vi "Main Window.vi"() -> ()   [LabVIEW 2020]
uses:
  Control Button/Exit.ctl
  Control Button/login.ctl
  Control Button/Logout.ctl
  Control Button/setting.ctl
  Control Button/report.ctl
  Control Button/Manual.ctl
  Control Button/Start.ctl
  Enqueue/Main window Seq/Test selection_1.ctl
  Enqueue/Main window Seq/Test seq_1.ctl
  Galobal variable_TI.vi
  Project Setup/Globle Variable/GR_Servo.vi
  <vilib>/Utility/file.llb/Read Delimited Spreadsheet (DBL).vi
panel:
  out "Boolean 3":bool
  in  "Boolean 2":bool
  out "Numeric 2":i32
  out "Company Name  2":string
  out "Error":bool
  out "User Name":string
  out "error out":errorcluster
  out "x = y?":bool
  out "Company Name":string
  in  "Sign In":T1
  out "Boolean":bool
  in  "Dashbord":T6
  in  "Login Window":T8 {"User Name" items=["admin", "mmum", "a", "AJAY Kumar", "", "", "", "", "", "", "", "", "", "", "", "", "", "", "", "", "", "", "", "", "", "", "", "", "", "", "", ""]}
  in  "Exit":T9
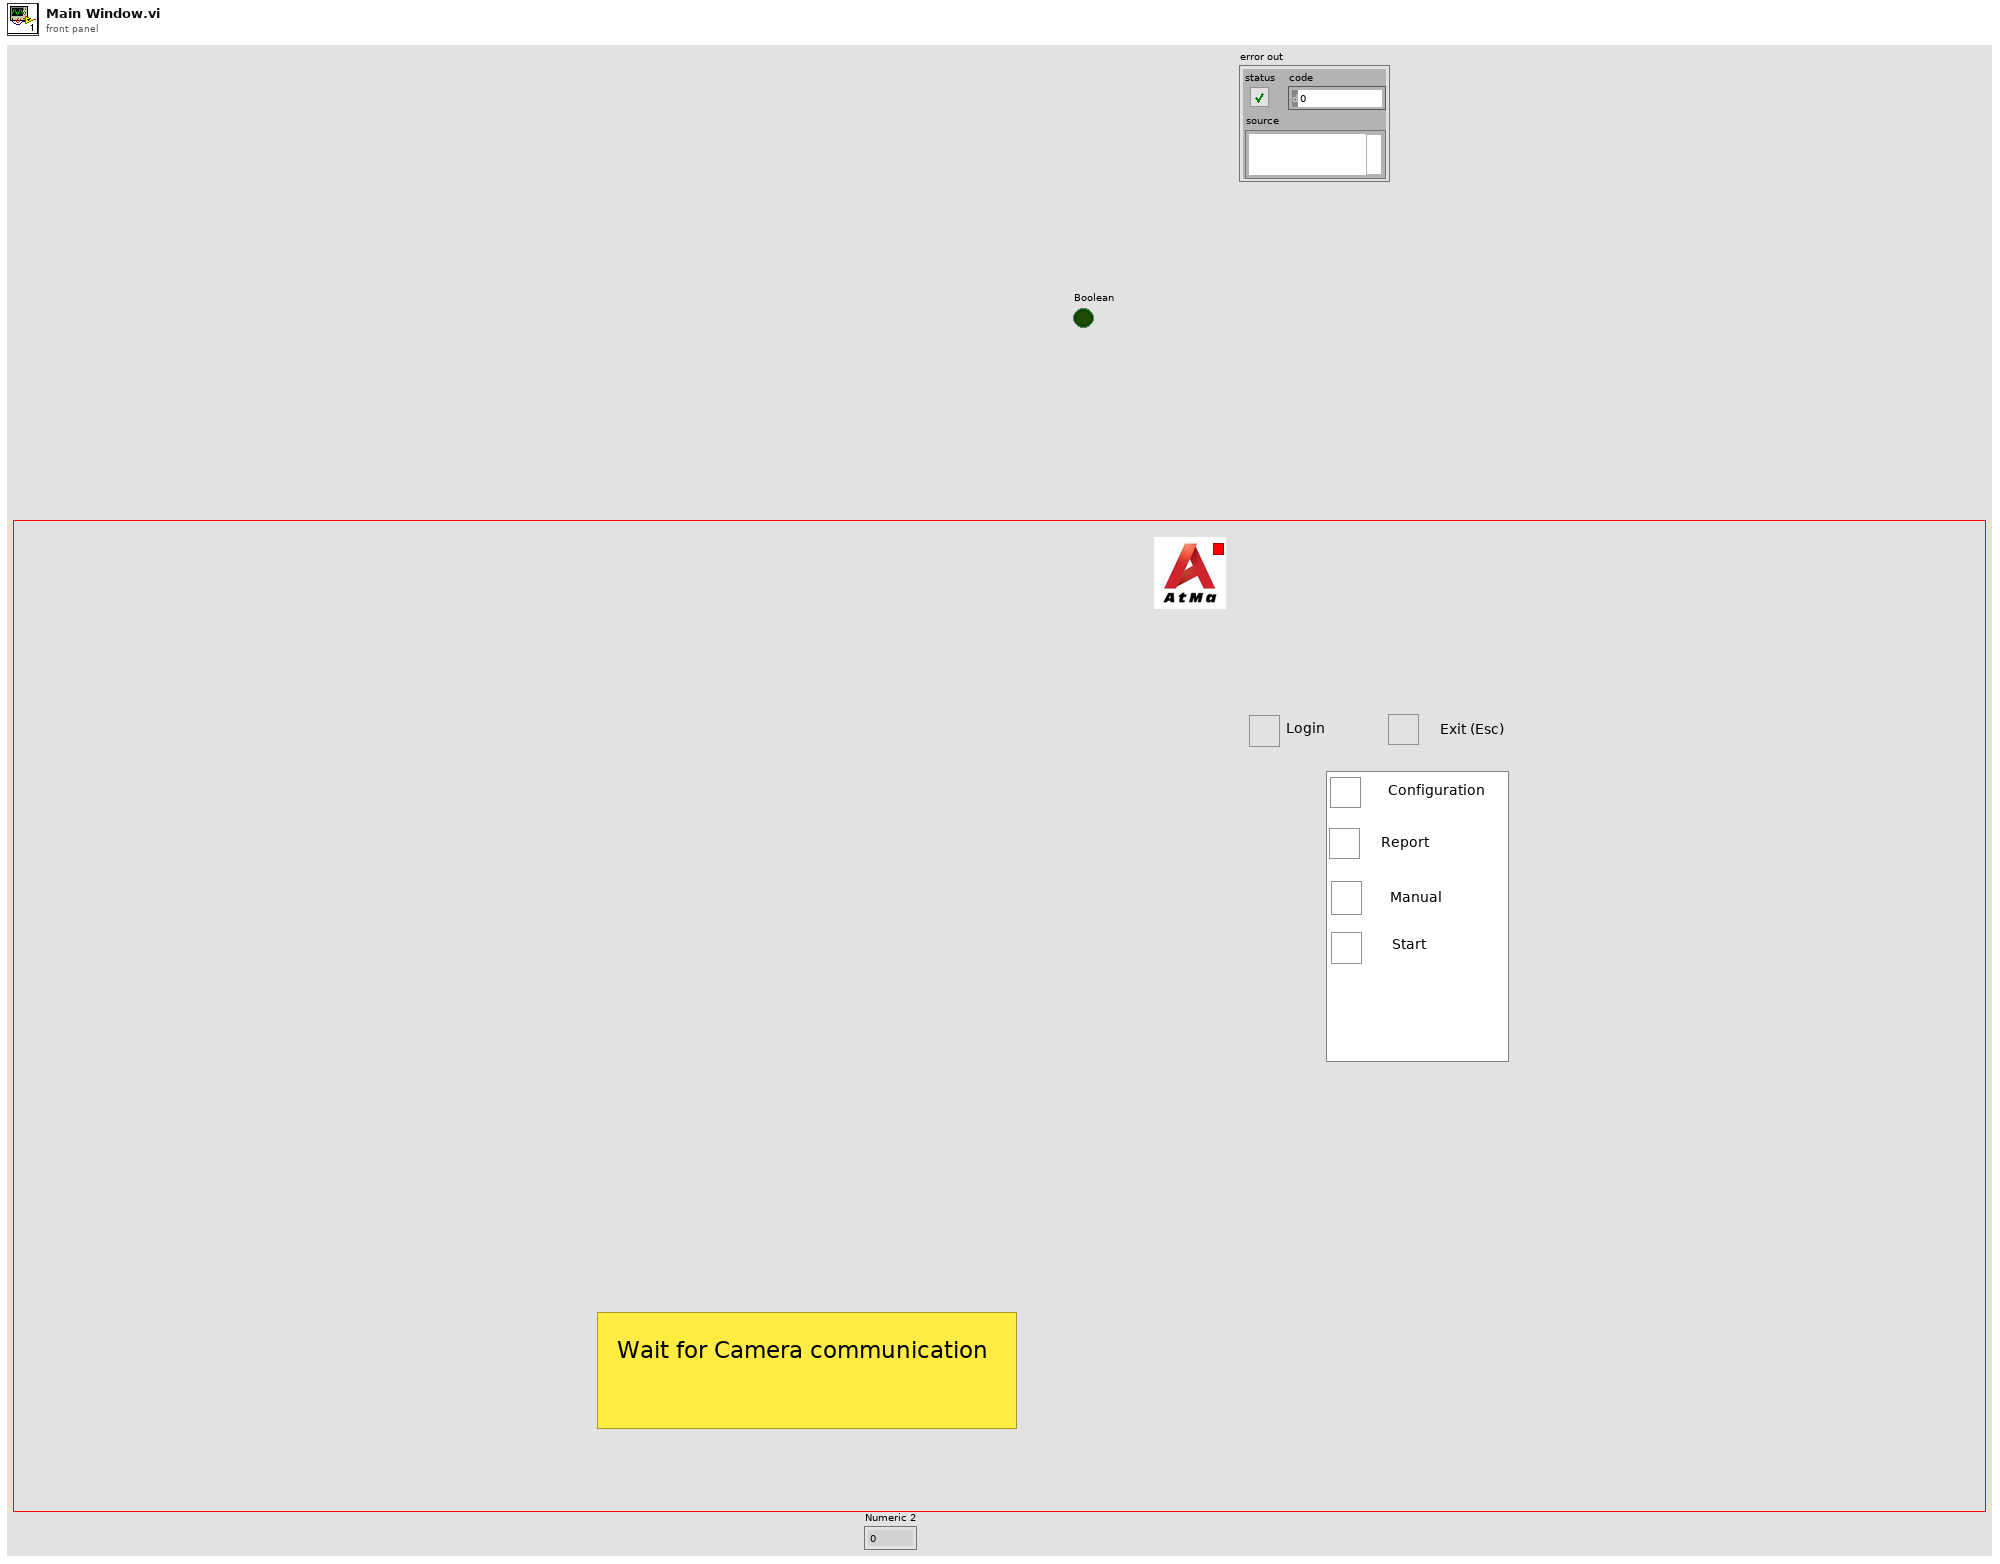
[diagram p1: front panel]
types:
  T1 = typedef "login.ctl" = bool
  T2 = typedef "setting.ctl" = bool
  T3 = typedef "report.ctl" = bool
  T4 = typedef "Manual.ctl" = bool
  T5 = typedef "Start.ctl" = bool
  T6 = cluster{"Setting":T2, "Report":T3, "Manaul":T4, "Start":T5}
  T7 = typedef "Logout.ctl" = bool
  T8 = cluster{"User Name":u16, "Password":string, "Sign In":T1, "Log Out":T7}
  T9 = typedef "Exit.ctl" = bool
  T10 = typedef "Test selection_1.ctl" = enum16{"Init", "Enqueue ", "Enqueue N", "Enqueue in stack", "Enqueue in stack N", "Dequeue", "Dequeue N", "Flush", "Release Queue"}
  T11 = typedef "Test seq_1.ctl" = enum16{"Poll Event", "Login", "Logout", "Confi", "Manual", "Report", "Testing", "Exit"}
  T12 = cluster{"XInput":dbl[], "Y New Value":dbl[], "Avg point":i16}[]
  T13 = cluster{"Slop":dbl[], "Intercept":dbl[], "Average ":i16[]}
  T14 = cluster{"UserName":string[], "Password":string[], "Usertype":string[], "Analog Min":string[], "Analog Max":string[], "DigitalInput Port":string[], "Digital Output Port":string[], "ANalog Port":string[], "IOList":cluster{"DI List_280":string[], "D0List _280":string[], "AI List_280":string[]}}
  T15 = cluster{"DI List_280":string[], "D0List _280":string[], "AI List_280":string[]}
  T16 = cluster{"DigitalInput Port[0]":string, "DigitalInput Port[1]":string, "DigitalInput Port[2]":string, "DigitalInput Port[3]":string, "DigitalInput Port[4]":string, "DigitalInput Port[5]":string, "DigitalInput Port[6]":string, "DigitalInput Port[7]":string, "DigitalInput Port[8]":string, "DigitalInput Port[9]":string, "DigitalInput Port[10]":string, "DigitalInput Port[11]":string, "DigitalInput Port[12]":string, "DigitalInput Port[13]":string, "DigitalInput Port[14]":string, "DigitalInput Port[15]":string}
  T17 = cluster{"Digital Output Port[0]":string, "Digital Output Port[1]":string, "Digital Output Port[2]":string, "Digital Output Port[3]":string, "Digital Output Port[4]":string, "Digital Output Port[5]":string, "Digital Output Port[6]":string, "Digital Output Port[7]":string, "Digital Output Port[8]":string, "Digital Output Port[9]":string, "Digital Output Port[10]":string, "Digital Output Port[11]":string, "Digital Output Port[12]":string, "Digital Output Port[13]":string, "Digital Output Port[14]":string, "Digital Output Port[15]":string, "Digital Output Port[16]":string, "Digital Output Port[17]":string, "Digital Output Port[18]":string, "Digital Output Port[19]":string, "Digital Output Port[20]":string, "Digital Output Port[21]":string, "Digital Output Port[22]":string, "Digital Output Port[23]":string, "Digital Output Port[24]":string, "Digital Output Port[25]":string, "Digital Output Port[26]":string, "Digital Output Port[27]":string, "Digital Output Port[28]":string, "Digital Output Port[29]":string}
  T18 = cluster{"ANalog Port[0]":string, "ANalog Port[1]":string, "ANalog Port[2]":string, "ANalog Port[3]":string, "ANalog Port[4]":string, "ANalog Port[5]":string, "ANalog Port[6]":string, "ANalog Port[7]":string, "ANalog Port[8]":string, "ANalog Port[9]":string, "ANalog Port[10]":string, "ANalog Port[11]":string, "ANalog Port[12]":string, "ANalog Port[13]":string, "ANalog Port[14]":string, "ANalog Port[15]":string, "ANalog Port[16]":string, "ANalog Port[17]":string, "ANalog Port[18]":string, "ANalog Port[19]":string, "ANalog Port[20]":string, "ANalog Port[21]":string, "ANalog Port[22]":string, "ANalog Port[23]":string, "ANalog Port[24]":string, "ANalog Port[25]":string, "ANalog Port[26]":string, "ANalog Port[27]":string, "ANalog Port[28]":string, "ANalog Port[29]":string, "ANalog Port[30]":string, "ANalog Port[31]":string}
  T19 = enum32{"Invalid", "Standard", "Closed", "Hidden", "Minimized", "Maximized"}
  T20 = enum8{"Enabled", "Disabled", "Disabled and Grayed Out"}
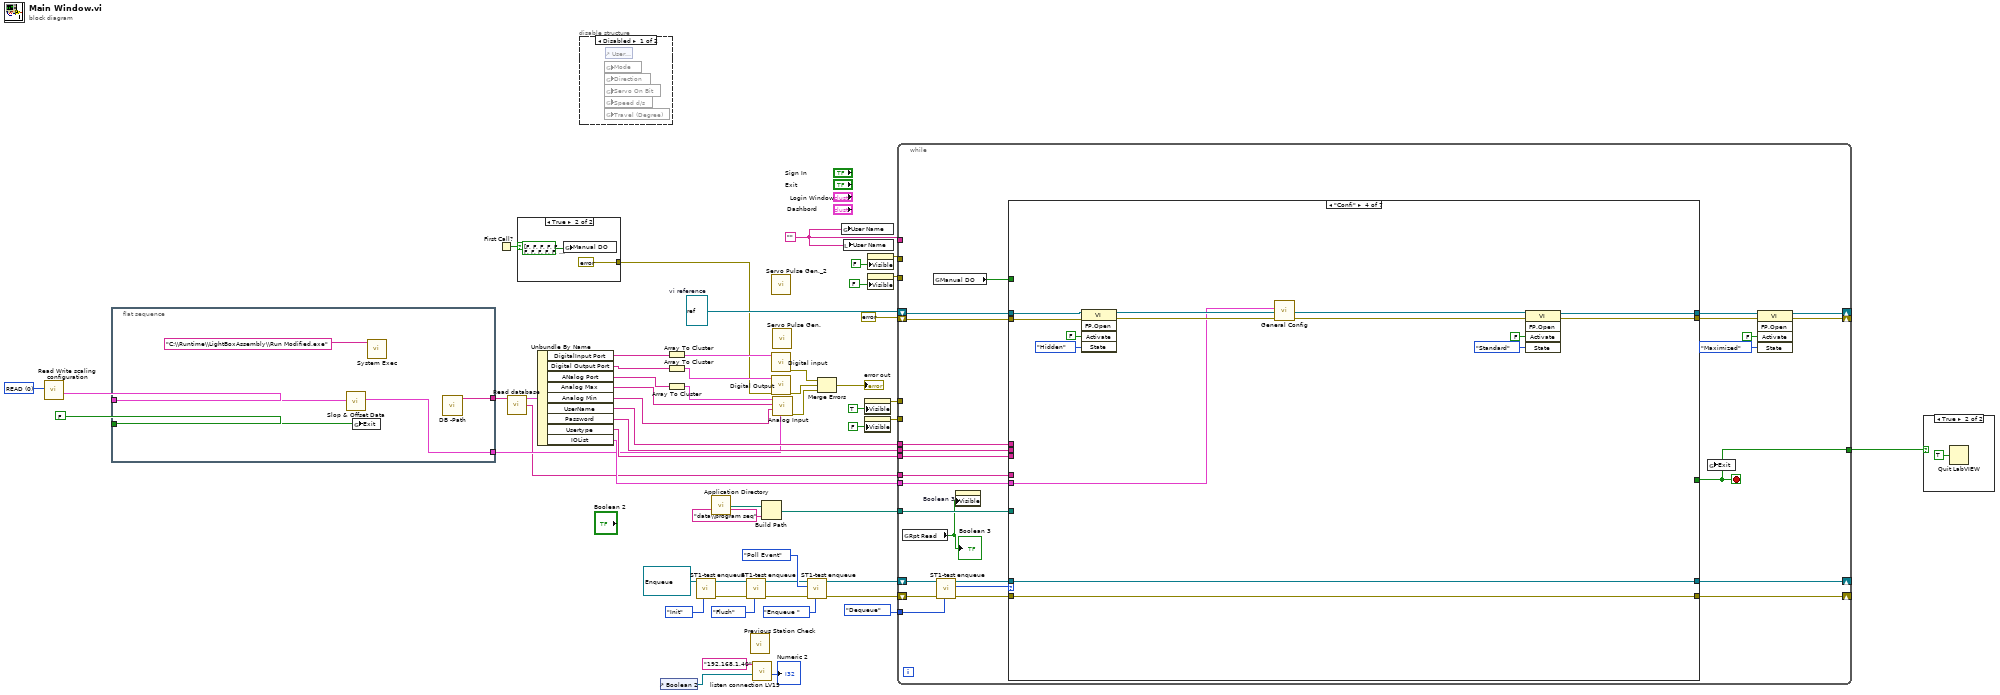
[diagram p0: block diagram]
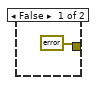
[diagram p3: hidden frame]
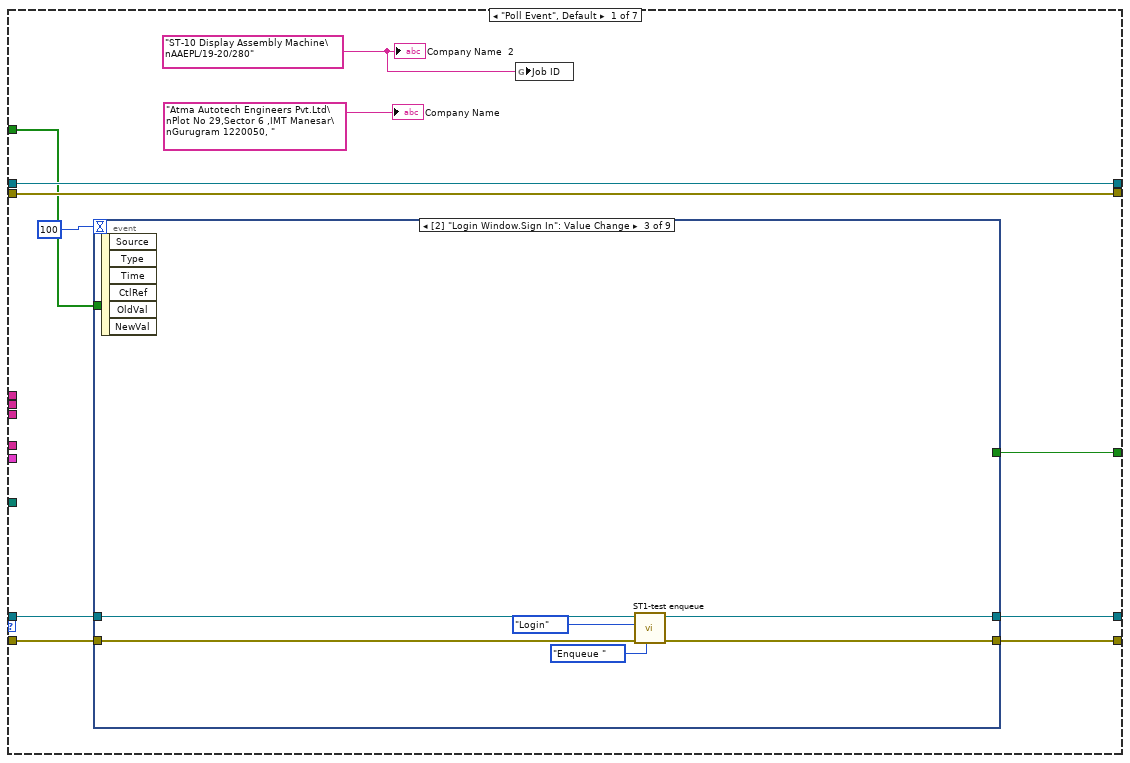
[diagram p5: hidden frame]
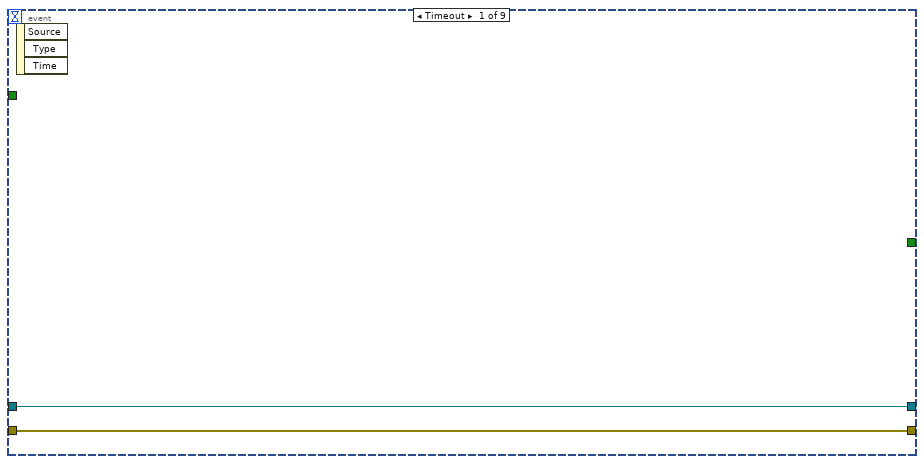
[diagram p6: hidden frame]
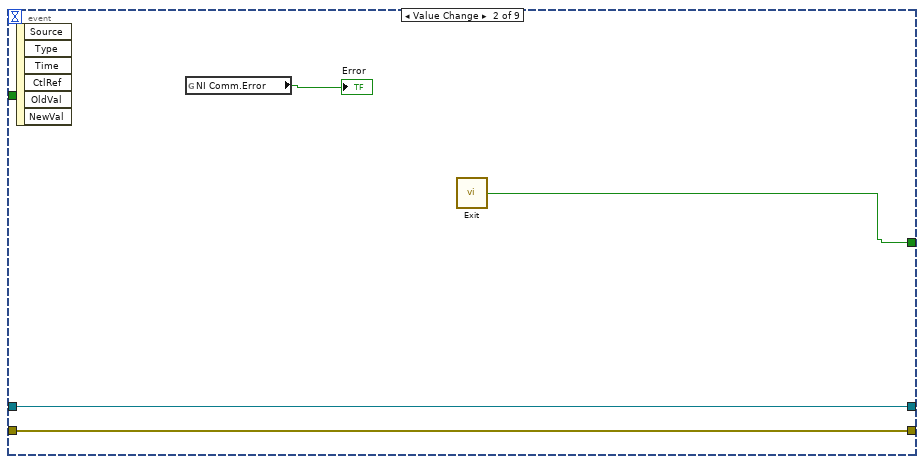
[diagram p7: hidden frame]
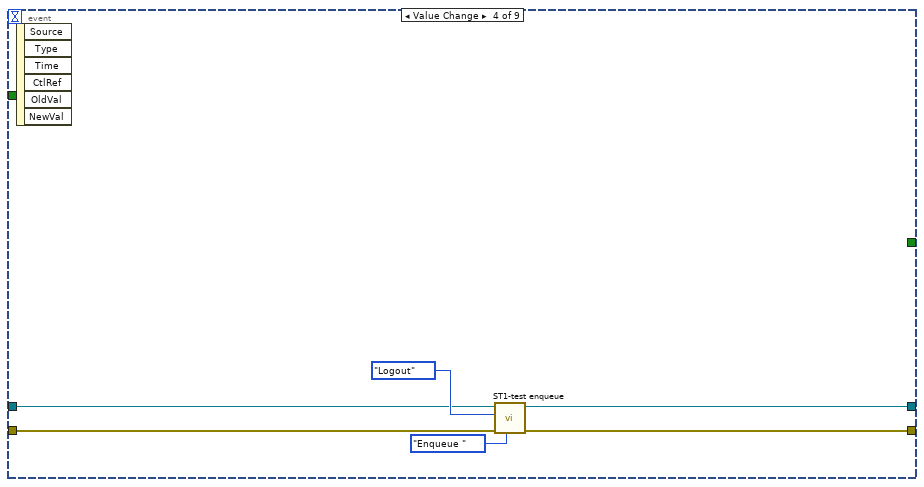
[diagram p8: hidden frame]
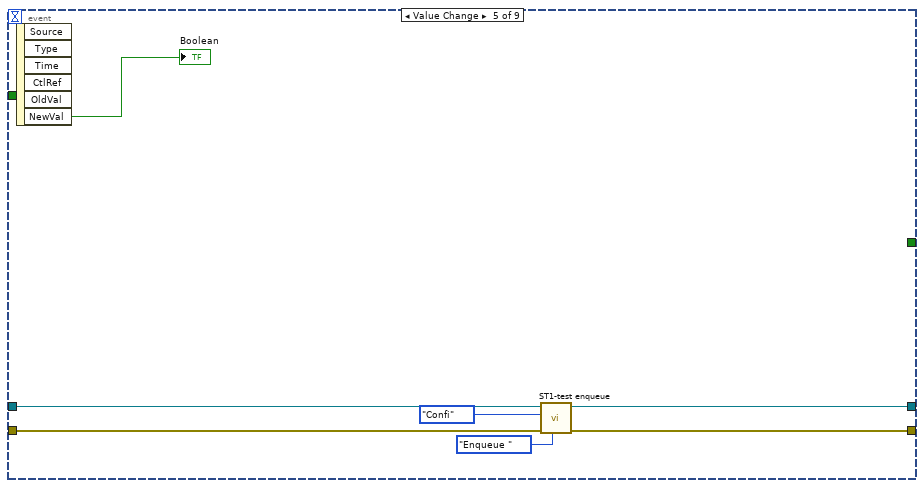
[diagram p9: hidden frame]
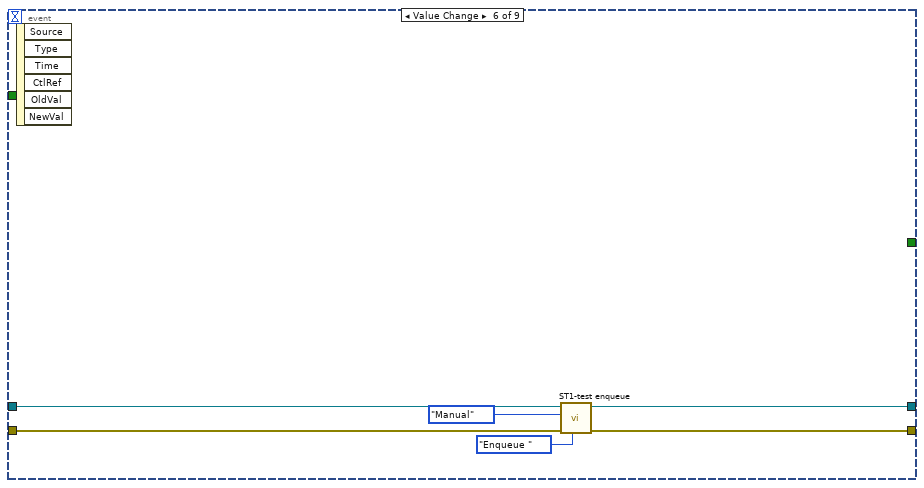
[diagram p10: hidden frame]
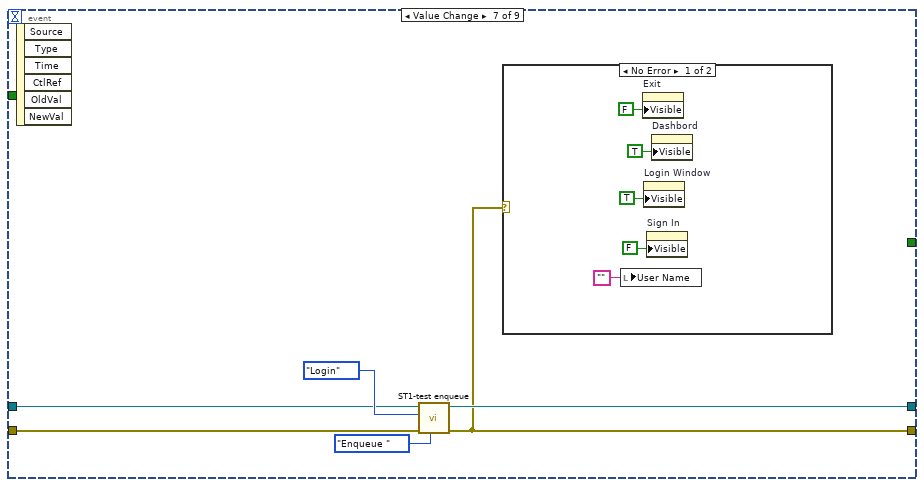
[diagram p11: hidden frame]
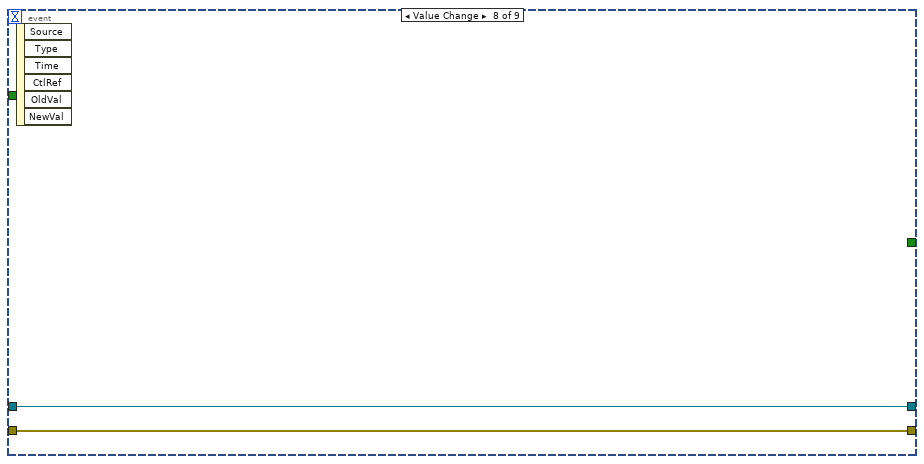
[diagram p13: hidden frame]
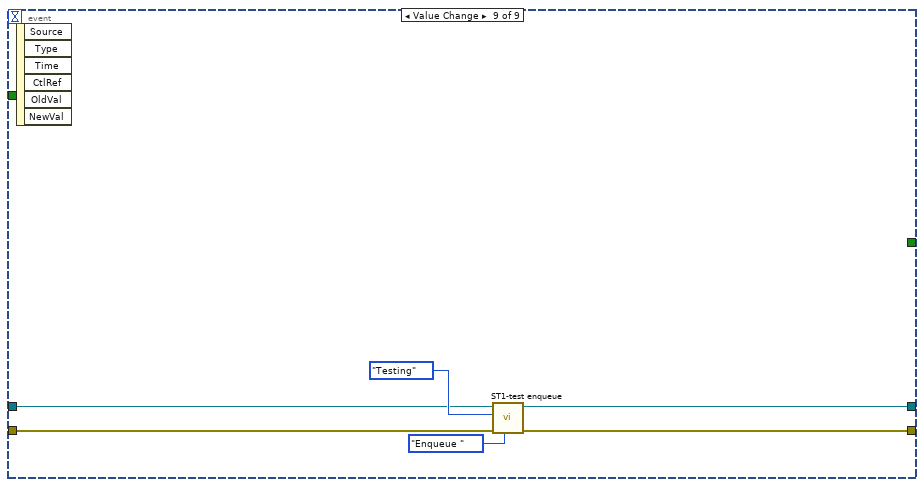
[diagram p14: hidden frame]
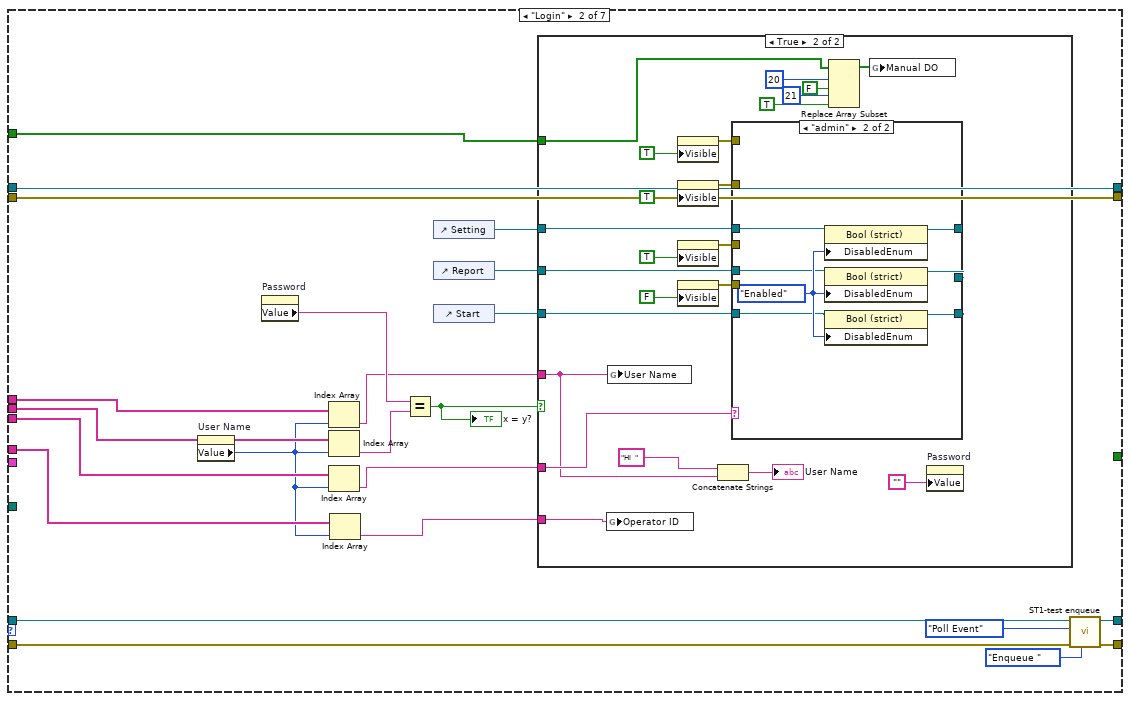
[diagram p15: hidden frame]
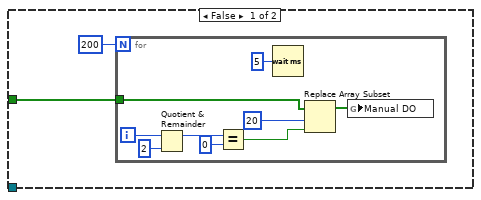
[diagram p16: hidden frame]
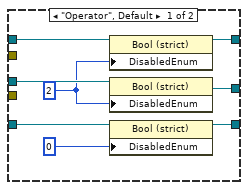
[diagram p17: hidden frame]
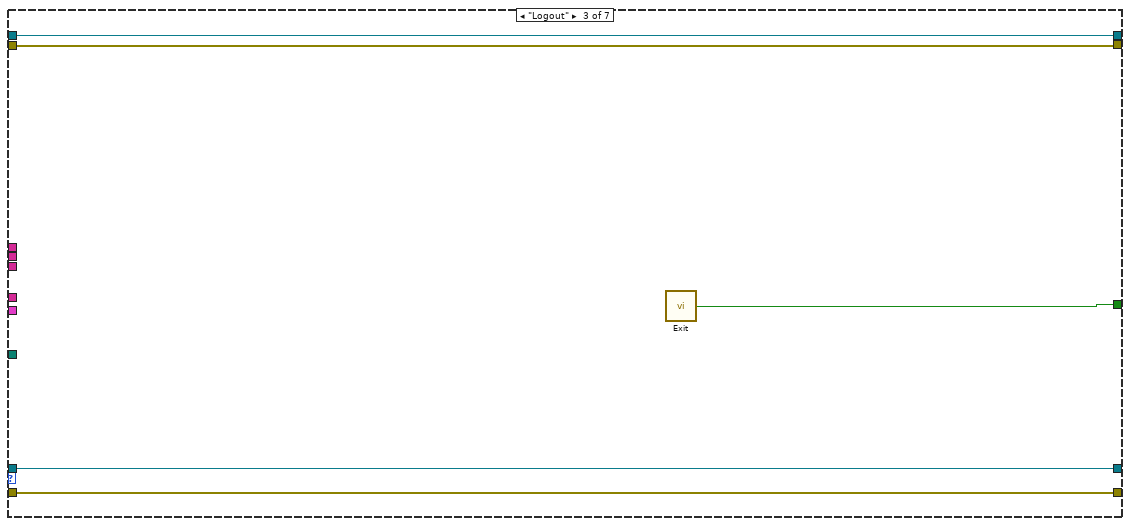
[diagram p18: hidden frame]
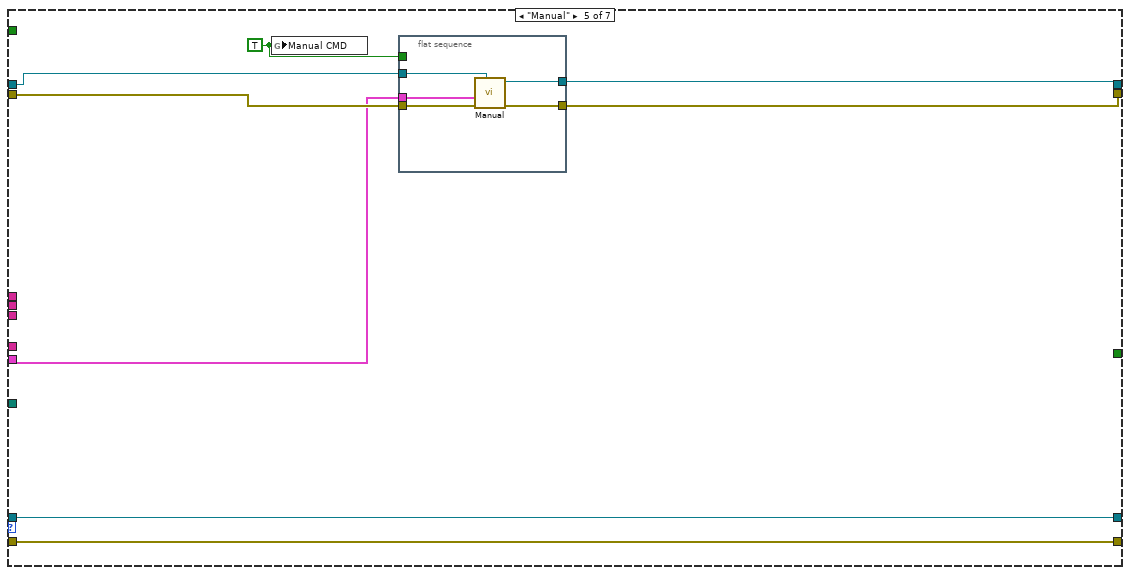
[diagram p19: hidden frame]
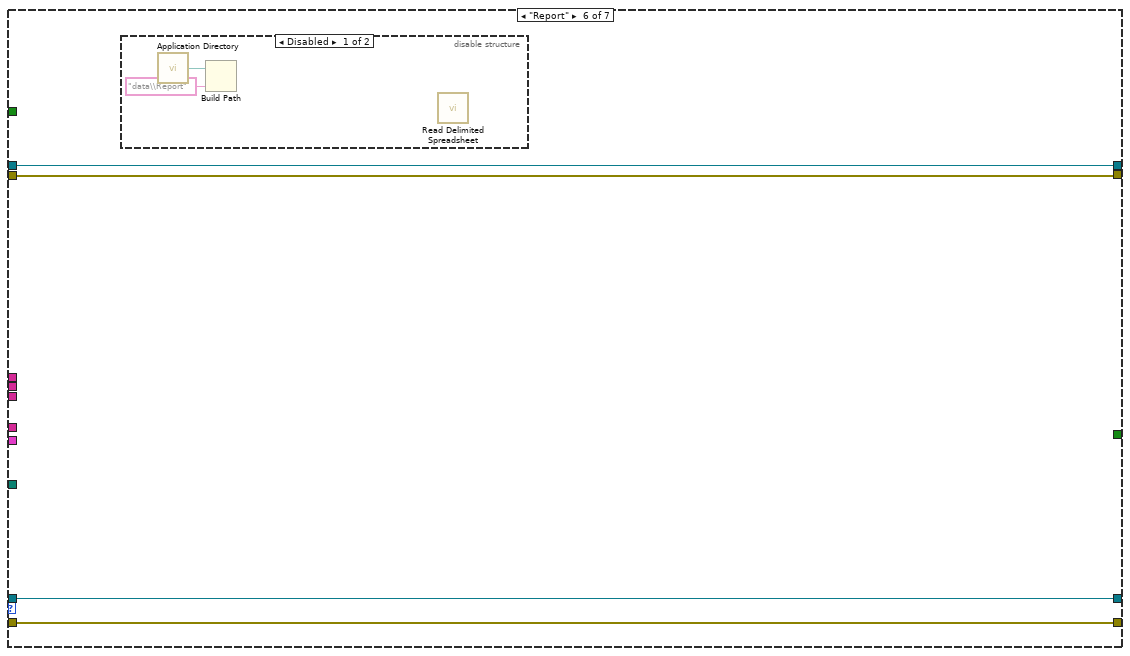
[diagram p20: hidden frame]
diagram:
  w18 = u16 0 items=["READ", "WRITE"] ("Read/Write")
  w33 = ""
  w43 = refnum<vi> refnum  # vi reference
  w44 = refnum<queue> refnum items=["Poll Event", "Login", "Logout", "Confi", "Manual", "Report", "Testing", "Exit"] ("queue in")
  n1 = call "Read Write scaling configuration.vi"("Read/Write"=w18) -> ("Output"=w17:T12)  [unwired: 4 in, 2 out]
  n2 = flat-sequence {
    tunnel: [w60] -> w32
    tunnel: w17 -> [w59]
    tunnel: [w58] -> w16
    tunnel: FALSE ("Exit") -> [w57]
    frame #0 {
      n3 = call "Slop & Offset Data.vi"("Input"=w59) -> ("Cluster"=w58:T13)  [unwired: 10 in]
      n4 = global write "Galobal variable_TI.vi" "Exit"(w57) -> ()
      n5 = call <vilib>:"System Exec.vi"("command line"="C:\\Runtime\\LightBoxAssembly\\Run Modified.exe") -> ()  [unwired: 7 in, 4 out]
      n6 = call "DB -Path.vi"() -> ("String"=w60:string)  [unwired: 11 in]
    }
  }
  n7 = First Call?() -> (First Call?: T/F=w7:bool)
  n8 = call "Read database.vi"("String"=w32) -> ("Operator Code"=w1:string[], "DB Data"=w31:T14)  [unwired: 2 in, 1 out]
  n9 = case shown="True" w7 {
    tunnel: [errorcluster {"status"=FALSE, "code"=0, "source"=""} ("error constant") errorcluster {"status"=FALSE, "code"=0, "source"=""} ("error constant")] -> w6
    frame False {
    }
    frame True {
      n10 = global write "Galobal variable_TI.vi" "Manual DO"(bool[] [FALSE, FALSE, FALSE, FALSE, FALSE, FALSE, FALSE, FALSE, FALSE, FALSE, FALSE, FALSE, FALSE, FALSE, FALSE, FALSE, FALSE, FALSE, FALSE, FALSE, FALSE, FALSE, FALSE, FALSE, FALSE, FALSE, FALSE, FALSE, FALSE, FALSE] ("Manual DO")) -> ()
    }
  }
  n11 = Unbundle By Name(w31) -> ("DigitalInput Port"=w30:string[], "Digital Output Port"=w28:string[], "ANalog Port"=w26:string[], "Analog Max"=w24:string[], "Analog Min"=w23:string[], "UserName"=w22:string[], "Password"=w21:string[], "Usertype"=w20:string[], "IOList"=w19:T15)
  n12 = disable-structure shown="Disabled" {
    frame Disabled {
      n13 = global read "GR_Servo.vi" "Mode"() -> ()  [unwired: 1 in]
      n14 = global read "GR_Servo.vi" "Direction"() -> ()  [unwired: 1 in]
      n15 = global read "GR_Servo.vi" "Servo On Bit"() -> ()  [unwired: 1 in]
      n16 = global read "GR_Servo.vi" "Speed d/s"() -> ()  [unwired: 1 in]
      n17 = global read "GR_Servo.vi" "Travel (Degree)"() -> ()  [unwired: 1 in]
      n18 = control-ref of="User Name"() -> ()  [unwired: 1 out]
    }
    frame Enabled {
    }
  }
  n19 = control-ref of="Boolean 2"() -> (w2:refnum<vi>)
  n20 = Array To Cluster(array=w30) -> (cluster=w29:T16)
  n21 = Array To Cluster(array=w28) -> (cluster=w27:T17)
  n22 = Array To Cluster(array=w26) -> (cluster=w25:T18)
  n23 = call "ST1-test enqueue.vi"("Enum Selection"=Test_selection_1."Init", "queue in"=w44) -> ("error out"=w53:errorcluster, "queue Out"=w49:refnum<queue>)  [unwired: 6 in, 1 out]
  n24 = call <vilib>:"Application Directory.vi"() -> ("Application Directory"=w10:path)
  n25 = call "ST1-test enqueue.vi"("Enum Selection"=Test_selection_1."Flush", "Error In"=w53, "queue in"=w49) -> ("error out"=w51:errorcluster, "queue Out"=w48:refnum<queue>)  [unwired: 5 in, 1 out]
  n26 = call "Previous Station Check.vi"() -> ()  [unwired: 12 in]
  n27 = call "listen connection LV15.vi"("Bool Refnum"=w2, "service name"="192.168.1.40") -> ("Numeric 2"=→"Numeric 2":i32)  [unwired: 6 in, 2 out]
  n28 = Build Path(base path=w10, name or relative path="data\\program seq") -> (appended path=w8:path)
  n29 = call "Digital Output.vi"("error in"=w6, "DAQmx OutPut Setting"=w27) -> ("error out"=w14:errorcluster)  [unwired: 8 in, 1 out]
  n30 = call "Servo Pulse Gen._2.vi"() -> ()  [unwired: 12 in]
  n31 = call "Digital input.vi"("DAQmx InPut Setting"=w29) -> ("error out"=w12:errorcluster)  [unwired: 9 in, 1 out]
  n32 = call "Servo Pulse Gen..vi"() -> ()  [unwired: 12 in]
  n33 = call "Analog Input.vi"("clai. Parmeter"=w16, "Min Value"=w23, "Max Value"=w24, "DAQmx Analog Input Setting"=w25) -> ("error out"=w13:errorcluster)  [unwired: 6 in, 1 out]
  n34 = call "ST1-test enqueue.vi"("Enum Selection"=Test_selection_1."Enqueue ", "Error In"=w51, "Enqueue"=Test_seq_1."Poll Event", "queue in"=w48) -> ("error out"=w46:errorcluster, "queue Out"=w47:refnum<queue>)  [unwired: 4 in, 1 out]
  n35 = Merge Errors(w12, w14, w13) -> (→"error out":errorcluster)
  n36 = global write "Galobal variable_TI.vi" "User Name"(w33) -> ()
  n37 = local write "User Name"(w33) -> ()
  n38 = property on="Login Window" class="Clust (strict)"("Visible"=TRUE) -> (error out=w38:errorcluster)  [unwired: 2 in, 1 out]
  n39 = property on="Sign In" class="Bool (strict)"("Visible"=FALSE) -> (error out=w37:errorcluster)  [unwired: 2 in, 1 out]
  n40 = property on="Exit" class="Bool (strict)"("Visible"=FALSE) -> (error out=w35:errorcluster)  [unwired: 2 in, 1 out]
  n41 = property on="Dashbord" class="Clust (strict)"("Visible"=FALSE) -> (error out=w40:errorcluster)  [unwired: 2 in, 1 out]
  n42 = while {
    shift-right: [w82] -> _
    shift-left: w47 -> [w88]
    shift-right: [w81] -> _
    shift-left: w46 -> [w87]
    tunnel: Test_selection_1."Dequeue" ("Enum Selection") -> [w86]
    shift-right: [w73] -> _
    shift-left: errorcluster {"status"=FALSE, "code"=0, "source"=""} ("error out") -> [w79]
    shift-right: [w74] -> _
    shift-left: w43 -> [w80]
    tunnel: w40 -> [_]
    tunnel: w38 -> [_]
    tunnel: w37 -> [_]
    tunnel: w35 -> [_]
    tunnel: w33 -> [_]
    tunnel: w22 -> [w72]
    tunnel: w21 -> [w71]
    tunnel: w20 -> [w70]
    tunnel: w19 -> [w69]
    tunnel: w8 -> [w68]
    tunnel: [w66] -> w5
    tunnel: w1 -> [w64]
    stop <- w66 stop-if-true
    n43 = global read "Galobal variable_TI.vi" "Rpt Read"() -> (w65:bool)
    "Boolean 3" <- w65
    n44 = global read "Galobal variable_TI.vi" "Manual DO"() -> (w67:bool[])
    n45 = call "ST1-test enqueue.vi"("Enum Selection"=w86, "Error In"=w87, "queue in"=w88) -> ("error out"=w83:errorcluster, "D-enqueue"=w85:T11, "queue Out"=w84:refnum<queue>)  [unwired: 5 in]
    n46 = property on="Boolean 3" class="Bool (strict)"("Visible"=w65) -> ()  [unwired: 2 in, 2 out]
    n47 = case shown="\"Confi\"" w85 {
      tunnel: [w97 _ w222 _ _ _ _] -> w66
      tunnel: w84 -> [w98 w154 w226 w240 w248 w257 w275]
      tunnel: w83 -> [w99 w153 w225 w239 w247 w256 w274]
      tunnel: [w96 w157 w226 w240 w248 w257 w275] -> w82
      tunnel: [w95 w156 w225 w239 w247 w256 w274] -> w81
      tunnel: [w94 w166 w224 w234 w243 w255 w262] -> w76
      tunnel: [w93 w165 w223 w233 w244 w254 w260] -> w75
      tunnel: w80 -> [w94 w166 w224 w232 w245 w255 w267]
      tunnel: w79 -> [w93 w165 w223 w231 w246 w254 w270]
      tunnel: w72 -> [_ w163 _ _ _ _ _]
      tunnel: w71 -> [_ w162 _ _ _ _ _]
      tunnel: w70 -> [_ w161 _ _ _ _ _]
      tunnel: w69 -> [_ _ _ w227 w242 _ w273]
      tunnel: w68 -> [_ _ _ _ _ _ w266]
      tunnel: w67 -> [w90 w155 _ _ _ _ _]
      tunnel: w64 -> [_ w152 _ _ _ _ _]
      frame "Poll Event", Default {
        w89 = "ST-10 Display Assembly Machine\nAAEPL/19-20/280" ("string")
        n48 = event shown="[2] \"Login Window.Sign In\": Value Change" {
          selector: _ -> [_ _ _ _ _ _ _ _ _]
          dyn-events: _ -> [_ _ _ _ _ _ _ _ _]
          timeout: 100 -> [_ _ _ _ _ _ _ _ _]
          tunnel: [_ w103 _ _ _ _ _ _ _] -> w97
          tunnel: w99 -> [w100 w104 w109 w112 w120 w128 w134 w142 w146]
          tunnel: w98 -> [w101 w105 w110 w113 w121 w126 w133 w143 w147]
          tunnel: [w101 w105 w108 w115 w119 w125 w132 w143 w145] -> w96
          tunnel: [w100 w104 w107 w114 w118 w127 w131 w142 w144] -> w95
          tunnel: w90 -> [_ _ _ _ _ _ _ _ _]
          event Timeout {
            n49 = event-data() -> ()  [unwired: 1 in, 3 out]
          }
          event Value Change {
            n50 = event-data() -> ()  [unwired: 1 in, 6 out]
            n51 = global read "Galobal variable_TI.vi" "NI Comm.Error"() -> (→"Error":bool)
            n52 = call "Exit.vi"() -> ("Exit"=w103:bool)  [unwired: 1 in]
          }
          event Value Change {
            n53 = event-data() -> ()  [unwired: 1 in, 6 out]
            n54 = call "ST1-test enqueue.vi"("Enum Selection"=Test_selection_1."Enqueue ", "Error In"=w109, "Enqueue"=Test_seq_1."Login", "queue in"=w110) -> ("error out"=w107:errorcluster, "queue Out"=w108:refnum<queue>)  [unwired: 4 in, 1 out]
          }
          event Value Change {
            n55 = event-data() -> ()  [unwired: 1 in, 6 out]
            n56 = call "ST1-test enqueue.vi"("Enum Selection"=Test_selection_1."Enqueue ", "Error In"=w112, "Enqueue"=Test_seq_1."Logout", "queue in"=w113) -> ("error out"=w114:errorcluster, "queue Out"=w115:refnum<queue>)  [unwired: 4 in, 1 out]
          }
          event Value Change {
            n57 = event-data() -> ("NewVal"=→"Boolean":T2)  [unwired: 1 in, 5 out]
            n58 = call "ST1-test enqueue.vi"("Enum Selection"=Test_selection_1."Enqueue ", "Error In"=w120, "Enqueue"=Test_seq_1."Confi", "queue in"=w121) -> ("error out"=w118:errorcluster, "queue Out"=w119:refnum<queue>)  [unwired: 4 in, 1 out]
          }
          event Value Change {
            n59 = event-data() -> ()  [unwired: 1 in, 6 out]
            n60 = call "ST1-test enqueue.vi"("Enum Selection"=Test_selection_1."Enqueue ", "Error In"=w128, "Enqueue"=Test_seq_1."Manual", "queue in"=w126) -> ("error out"=w127:errorcluster, "queue Out"=w125:refnum<queue>)  [unwired: 4 in, 1 out]
          }
          event Value Change {
            n61 = event-data() -> ()  [unwired: 1 in, 6 out]
            n62 = call "ST1-test enqueue.vi"("Enum Selection"=Test_selection_1."Enqueue ", "Error In"=w134, "Enqueue"=Test_seq_1."Login", "queue in"=w133) -> ("error out"=w131:errorcluster, "queue Out"=w132:refnum<queue>)  [unwired: 4 in, 1 out]
            n63 = case shown="No Error" w131 {
              frame No Error {
                n64 = local write "User Name"("") -> ()
                n65 = property on="Exit" class="Bool (strict)"("Visible"=FALSE) -> ()  [unwired: 2 in, 2 out]
                n66 = property on="Login Window" class="Clust (strict)"("Visible"=TRUE) -> ()  [unwired: 2 in, 2 out]
                n67 = property on="Sign In" class="Bool (strict)"("Visible"=FALSE) -> ()  [unwired: 2 in, 2 out]
                n68 = property on="Dashbord" class="Clust (strict)"("Visible"=TRUE) -> ()  [unwired: 2 in, 2 out]
              }
              frame Error {
              }
            }
          }
          event Value Change {
            n69 = event-data() -> ()  [unwired: 1 in, 6 out]
          }
          event Value Change {
            n70 = event-data() -> ()  [unwired: 1 in, 6 out]
            n71 = call "ST1-test enqueue.vi"("Enum Selection"=Test_selection_1."Enqueue ", "Error In"=w146, "Enqueue"=Test_seq_1."Testing", "queue in"=w147) -> ("error out"=w144:errorcluster, "queue Out"=w145:refnum<queue>)  [unwired: 4 in, 1 out]
          }
        }
        n72 = global write "Galobal variable_TI.vi" "Job ID"(w89) -> ()
        "Company Name" <- "Atma Autotech Engineers Pvt.Ltd\nPlot No 29,Sector 6 ,IMT Manesar\nGurugram 1220050, " ("string")
        "Company Name  2" <- w89
      }
      frame "Login" {
        n73 = property on="User Name" class="Ring (strict)"() -> ("Value"=w151:u16)  [unwired: 2 in, 2 out]
        n74 = property on="Password" class="Str"() -> ("Value"=w171:string)  [unwired: 2 in, 2 out]
        n75 = Index Array(array=w163, index=w151) -> (element=w164:string)
        n76 = Index Array(array=w162, index=w151) -> (element=w172:string)
        n77 = Index Array(array=w161, index=w151) -> (element=w170:string)
        n78 = Index Array(array=w152, index=w151) -> (element=w150:string)
        n79 = Equal?(x=w171, y=w172) -> (x = y?=w160:bool)
        "x = y?" <- w160
        n80 = control-ref of="Setting"() -> (w169:refnum<vi>)
        n81 = control-ref of="Report"() -> (w167:refnum<vi>)
        n82 = control-ref of="Start"() -> (w168:refnum<vi>)
        n83 = case shown="True" w160 {
          tunnel: w170 -> [_ w202]
          tunnel: w169 -> [_ w206]
          tunnel: w167 -> [_ w205]
          tunnel: w168 -> [_ w204]
          tunnel: w164 -> [_ w185]
          tunnel: w155 -> [w173 w189]
          tunnel: w150 -> [_ w184]
          frame False {
            n84 = for {
              N: 200 -> [_]
              tunnel: w173 -> [w175]
              i -> [w183]
              n85 = Quotient & Remainder(x=w183, y=2) -> (x-y*floor(x/y)=w181:i32)  [unwired: 1 out]
              n86 = Equal?(x=w181, y=0) -> (x = y?=w178:bool)
              n87 = Wait (ms)(milliseconds to wait=u32 5) -> ()  [unwired: 1 out]
              n88 = Replace Array Subset(array=w175, new element=w178, index=20) -> (w176:bool[])
              n89 = global write "Galobal variable_TI.vi" "Manual DO"(w176) -> ()
            }
          }
          frame True {
            n90 = global write "Galobal variable_TI.vi" "Operator ID"(w184) -> ()
            n91 = global write "Galobal variable_TI.vi" "User Name"(w185) -> ()
            n92 = property on="Exit" class="Bool (strict)"("Visible"=TRUE) -> (error out=w193:errorcluster)  [unwired: 2 in, 1 out]
            n93 = property on="Dashbord" class="Clust (strict)"("Visible"=TRUE) -> (error out=w198:errorcluster)  [unwired: 2 in, 1 out]
            n94 = property on="Sign In" class="Bool (strict)"("Visible"=TRUE) -> (error out=w197:errorcluster)  [unwired: 2 in, 1 out]
            n95 = property on="Login Window" class="Clust (strict)"("Visible"=FALSE) -> (error out=w199:errorcluster)  [unwired: 2 in, 1 out]
            n96 = Concatenate Strings("Hi  " ("string"), w185) -> (→"User Name":string)
            n97 = case shown="\"admin\"" w202 {
              tunnel: [w214 w220] -> _
              tunnel: [w213 w219] -> _
              tunnel: [w212 w218] -> _
              tunnel: w206 -> [w211 w217]
              tunnel: w205 -> [w210 w216]
              tunnel: w204 -> [w209 w215]
              tunnel: w199 -> [_ _]
              tunnel: w198 -> [_ _]
              tunnel: w197 -> [_ _]
              tunnel: w193 -> [_ _]
              frame "Operator", Default {
                w207 = 2
                n98 = property class="Bool (strict)"(reference=w211, "DisabledEnum"=w207) -> (reference out=w214:refnum<vi>)  [unwired: 1 in, 1 out]
                n99 = property class="Bool (strict)"(reference=w210, "DisabledEnum"=w207) -> (reference out=w213:refnum<vi>)  [unwired: 1 in, 1 out]
                n100 = property class="Bool (strict)"(reference=w209, "DisabledEnum"=0) -> (reference out=w212:refnum<vi>)  [unwired: 1 in, 1 out]
              }
              frame "admin" {
                w221 = T20."Enabled" ("Disabled")
                n101 = property class="Bool (strict)"(reference=w217, "DisabledEnum"=w221) -> (reference out=w220:refnum<vi>)  [unwired: 1 in, 1 out]
                n102 = property class="Bool (strict)"(reference=w216, "DisabledEnum"=w221) -> (reference out=w219:refnum<vi>)  [unwired: 1 in, 1 out]
                n103 = property class="Bool (strict)"(reference=w215, "DisabledEnum"=w221) -> (reference out=w218:refnum<vi>)  [unwired: 1 in, 1 out]
              }
            }
            n104 = Replace Array Subset(array=w189, new element #1=FALSE ("new element/subarray"), index #1=20 ("index"), new element #2=TRUE ("new element/subarray"), index #2=21 ("index")) -> (w190:bool[])
            n105 = global write "Galobal variable_TI.vi" "Manual DO"(w190) -> ()
            n106 = property on="Password" class="Str"("Value"="") -> ()  [unwired: 2 in, 2 out]
          }
        }
        n107 = call "ST1-test enqueue.vi"("Enum Selection"=Test_selection_1."Enqueue ", "Error In"=w153, "Enqueue"=Test_seq_1."Poll Event", "queue in"=w154) -> ("error out"=w156:errorcluster, "queue Out"=w157:refnum<queue>)  [unwired: 4 in, 1 out]
      }
      frame "Logout" {
        n108 = call "Exit.vi"() -> ("Exit"=w222:bool)  [unwired: 1 in]
      }
      frame "Confi" {
        n109 = invoke class="VI" method="FP.Open"(reference=w232, error in=w231, "Activate"=FALSE ("Activate?"), "State"=T19."Hidden") -> (reference out=w228:refnum<vi>, error out=w230:errorcluster)  [unwired: 1 in, 3 out]
        n110 = call "General Config.vi"("error In"=w230, "IOList"=w227) -> ("error out"=w229:errorcluster)  [unwired: 8 in, 1 out]
        n111 = invoke class="VI" method="FP.Open"(reference=w228, error in=w229, "Activate"=FALSE ("Activate?"), "State"=T19."Standard") -> (reference out=w234:refnum<vi>, error out=w233:errorcluster)  [unwired: 1 in, 3 out]
      }
      frame "Manual" {
        w241 = TRUE ("Manual CMD")
        n112 = global write "Galobal variable_TI.vi" "Manual CMD"(w241) -> ()
        n113 = flat-sequence {
          tunnel: w246 -> [w253]
          tunnel: w245 -> [w252]
          tunnel: [w251] -> w244
          tunnel: [w250] -> w243
          tunnel: w242 -> [w249]
          tunnel: w241 -> [_]
          frame #0 {
            n114 = call "Manual.vi"("vi reference"=w252, "error in (no error)"=w253, "IOList_280"=w249) -> ("error out"=w251:errorcluster, "Out reference"=w250:refnum<vi>)  [unwired: 7 in]
          }
        }
      }
      frame "Report" {
        n115 = disable-structure shown="Disabled" {
          frame Disabled {
            n116 = call <vilib>:"Application Directory.vi"() -> ("Application Directory"=w259:path)
            n117 = Build Path(base path=w259, name or relative path="data\\Report") -> ()  [unwired: 1 out]
            n118 = call-poly <vilib>:"Read Delimited Spreadsheet.vi"() -> ()  [unwired: 10 in, 6 out]
          }
          frame Enabled {
          }
        }
      }
      frame "Testing" {
        n119 = Unbundle By Name(w273) -> ()  [unwired: 1 out]
        n120 = invoke class="VI" method="FP.Open"(reference=w267, error in=w270, "Activate"=FALSE ("Activate?"), "State"=T19."Hidden") -> (reference out=w269:refnum<vi>, error out=w268:errorcluster)  [unwired: 1 in, 3 out]
        n121 = call "Program list Selection.vi"("error in"=w268, "Filepath"=w266, "vi referenceIn"=w269) -> ("error out"=w261:errorcluster, "vi reference Out"=w263:refnum<vi>)  [unwired: 5 in, 2 out]
        n122 = invoke class="VI" method="FP.Open"(reference=w263, error in=w261, "Activate"=FALSE ("Activate?"), "State"=T19."Standard") -> (reference out=w262:refnum<vi>, error out=w260:errorcluster)  [unwired: 1 in, 3 out]
      }
    }
    n123 = global write "Galobal variable_TI.vi" "Exit"(w66) -> ()
    n124 = invoke class="VI" method="FP.Open"(reference=w76, error in=w75, "Activate"=FALSE ("Activate?"), "State"=T19."Maximized") -> (reference out=w74:refnum<vi>, error out=w73:errorcluster)  [unwired: 1 in, 3 out]
  }
  n125 = case shown="True" w5 {
    frame False {
    }
    frame True {
      n126 = Quit LabVIEW(quit? (T)=TRUE) -> ()
    }
  }
